vi "Pressure Temperature Monitor v3.vi"() -> ()   [LabVIEW 2016]
panel:
  in  "Gain":dbl=-10.0 format="%#_13g"
  in  "?":i32(ring)=2 items=["MKS 943 Cold Cathode"=1, "Thyracont All Range"=2]
  out "Pressure CH3":dbl=0.0007462942310144351 format="%#.2e"
  out "PRE Pressure 2":dbl(graph)=0.0007462942310144351
  in  "Gain":dbl=-10.0 format="%#_13g"
  in  "?":i32(ring)=1 items=["MKS 943 Cold Cathode"=1, "Thyracont All Range"=2]
  in  "?":i32(ring)=1 items=["MKS 943 Cold Cathode"=1, "Thyracont All Range"=2]
  in  "?":bool
  out "Pressure CH2":dbl=1.0051507111908389e-10 format="%#.2e"
  out "LL Pressure":dbl(graph)=1.0051507111908389e-10
  out "Tempreture CH2":dbl=3407.210278151436 format="%.1f"
  out "T2 Tempreture":dbl(graph)=3407.210278151436
  in  "Gain":dbl=-10.0 format="%#_13g"
  out "Tempreture CH1":dbl=21.38127177176258 format="%.1f"
  out "Pressure CH1":dbl=1.7008193334756893e-10 format="%#.2e"
  out "Heater Tempreture":dbl(graph)=21.38127177176258
  in  "?":bool
  out "Overdosing":bool
  in  "Dosing Limit":dbl=20.0 format="%#.2f"
  in  "Base Pressure":dbl=1e-10 format="%#.2e"
  out "PRE Pressure":dbl(graph)=1.7008193334756893e-10
  out "L":dbl=0.0047677960618811325 format="%.1e"
  in  "Pressure Limit":dbl=10.0 format="%#.2e"
  in  "?":bool
  # "Prep Pressure (Torr)"
  # "STM Pressure"
  # "LL Pressure"
  # "(Torr)"
  # "(Torr)"
  # "(Torr)"
  # "CH1 Temperature"
  # "CH2 Temperature"
  # "Langmuir"
  # "(°C )"
  # "(°C )"
  # "STM"
  # "PRE"
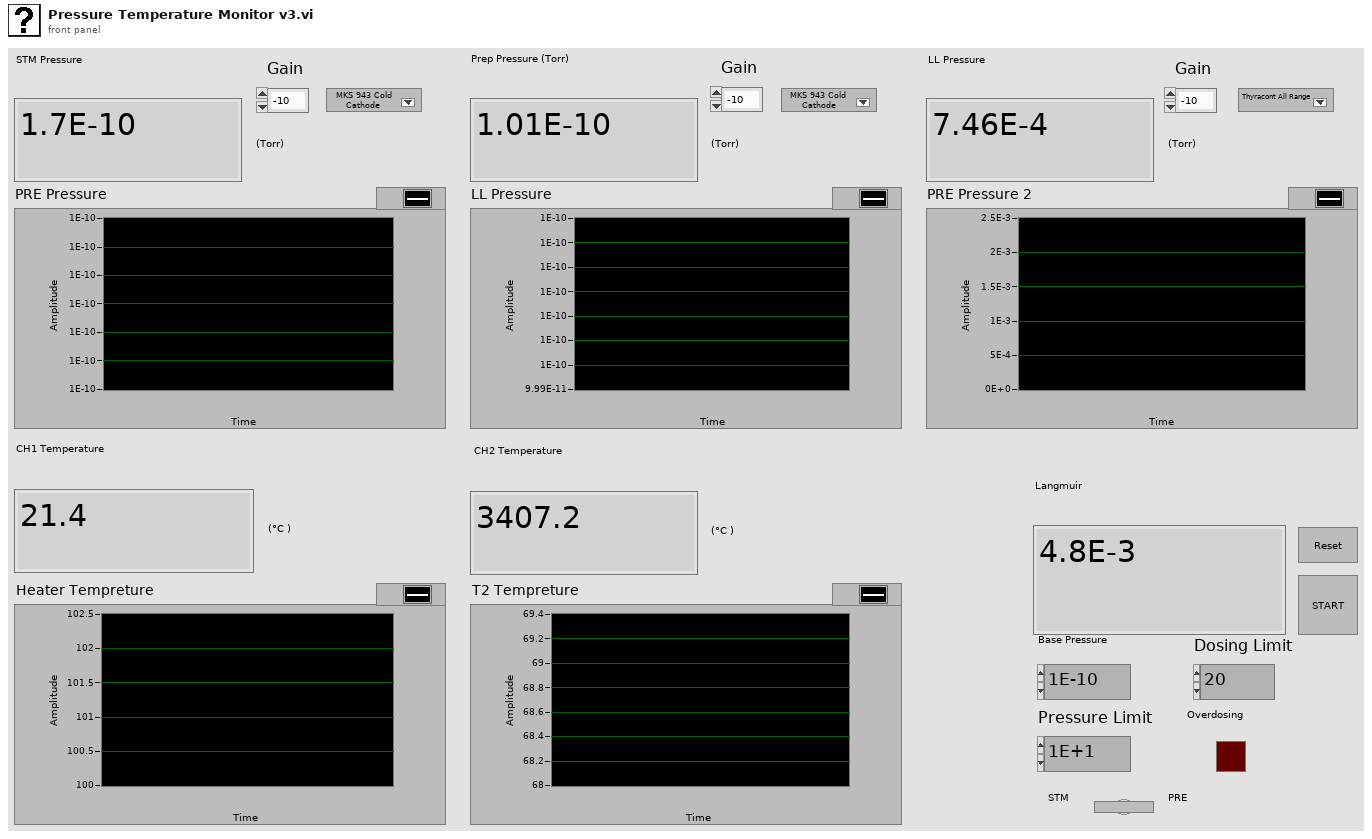
[diagram p1: front panel]
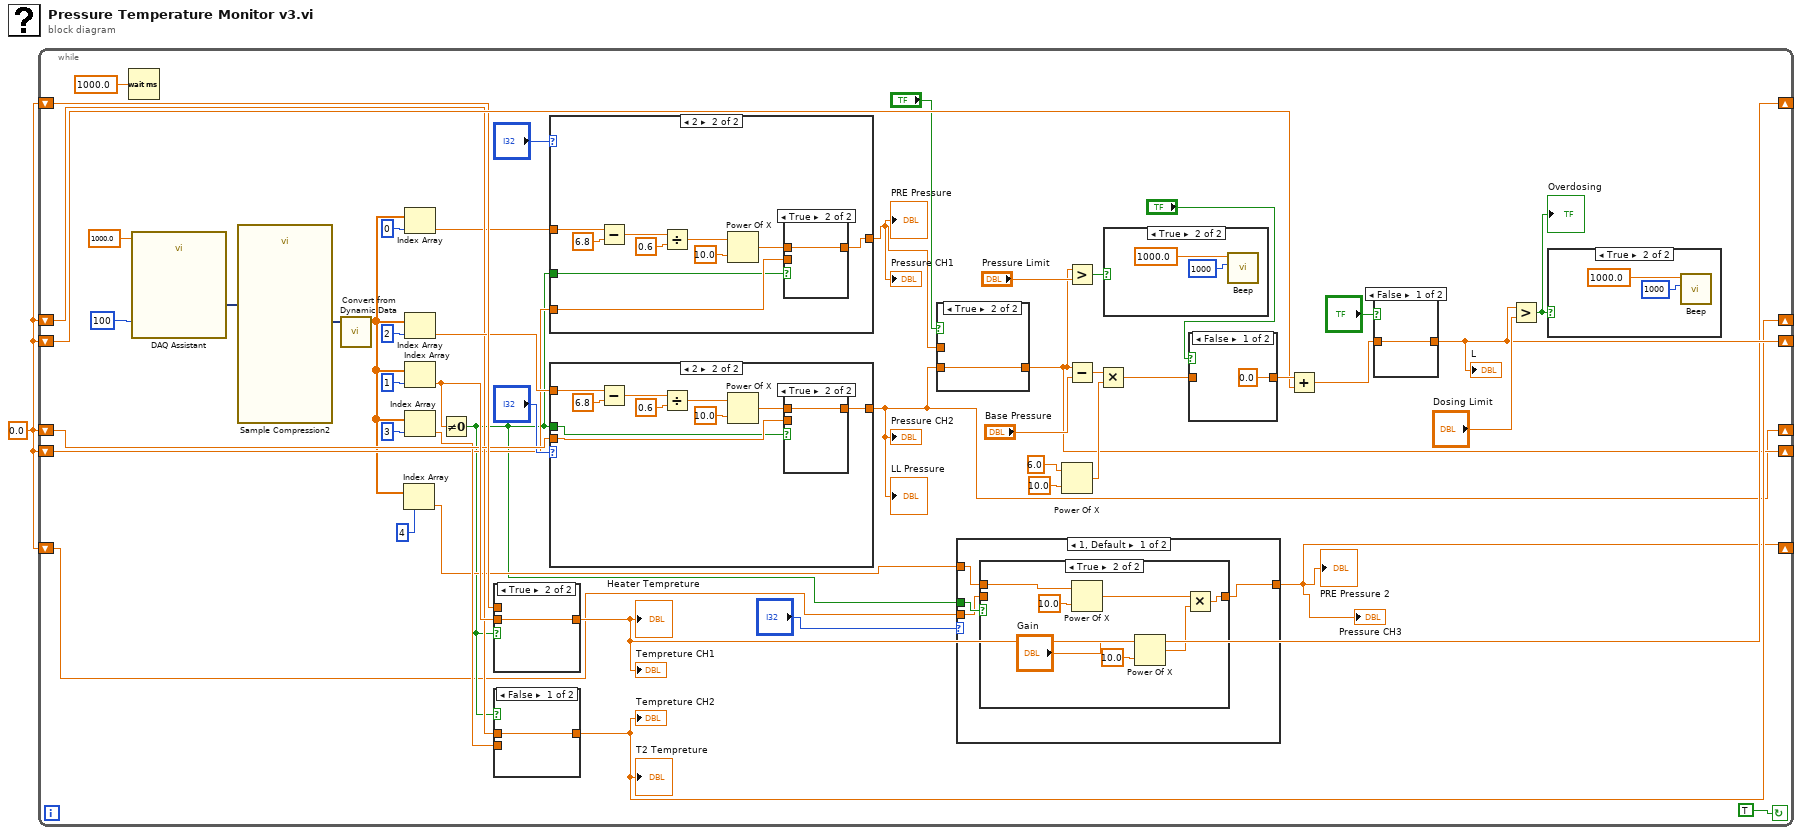
[diagram p0: block diagram]
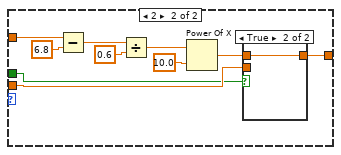
[diagram p3: hidden frame]
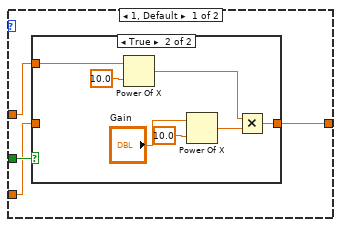
[diagram p5: hidden frame]
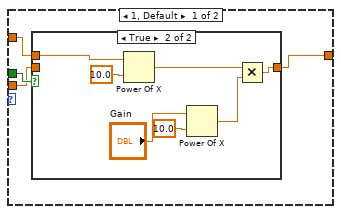
[diagram p8: hidden frame]
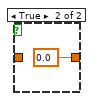
[diagram p14: hidden frame]
diagram:
  w1 = 0.0
  n1 = while {
    shift-left: w1 -> [w41]
    shift-right: [w39] -> _
    shift-right: [w15] -> _
    shift-left: w1 -> [w10]
    shift-right: [w33] -> _
    shift-left: w1 -> [w35]
    shift-right: [w13] -> _
    shift-left: w1 -> [w20]
    shift-right: [w17] -> _
    shift-left: w1 -> [w18]
    shift-right: [w2] -> _
    shift-left: w1 -> [w3]
    stop <- TRUE continue-if-true
    n2 = Wait (ms)(milliseconds to wait=1000.0 ("y")) -> ()  [unwired: 1 out]
    n3 = call "DAQ Assistant"("rate"=1000.0, "number of samples"=100) -> ("data"=w25:dynamicdata)  [unwired: 15 in, 2 out]
    n4 = call "Sample Compression2"("Signals"=w25) -> ("Mean"=w22:dynamicdata)  [unwired: 8 in, 2 out]
    n5 = call "Convert from Dynamic Data"("Dynamic Data Type"=w22) -> ("Array"=w7:dbl[])  [unwired: 3 in]
    n6 = Index Array(array=w7, index=4) -> (element=w6:dbl)
    n7 = Index Array(array=w7, index=0) -> (element=w12:dbl)
    n8 = Index Array(array=w7, index=2) -> (element=w21:dbl)
    n9 = Index Array(array=w7, index=1) -> (element=w34:dbl)
    n10 = Index Array(array=w7, index=3) -> (element=w19:dbl)
    n11 = Not Equal To 0?(x=w34) -> (x != 0?=w5:bool)
    n12 = case shown="True" w5 {
      tunnel: w34 -> [_ w128]
      tunnel: [w127 w128] -> w33
      tunnel: w35 -> [w127 _]
      frame False {
      }
      frame True {
      }
    }
    "Heater Tempreture" <- w33
    "Tempreture CH1" <- w33
    n13 = case shown="False" w5 {
      tunnel: w18 -> [w125 _]
      tunnel: [w125 w126] -> w17
      tunnel: w19 -> [_ w126]
      frame False {
      }
      frame True {
      }
    }
    "T2 Tempreture" <- w17
    "Tempreture CH2" <- w17
    n14 = case shown="2" "?" {
      tunnel: w5 -> [w78 w89]
      tunnel: w12 -> [w77 w88]
      tunnel: w10 -> [w76 w92]
      tunnel: [w75 w87] -> w9
      frame 1, Default {
        n15 = case shown="True" w78 {
          tunnel: w77 -> [_ w85]
          tunnel: [w79 w86] -> w75
          tunnel: w76 -> [w79 _]
          frame False {
          }
          frame True {
            n16 = Power Of X(1:10.0 ("x"), 2:w85) -> (0:w84:dbl)
            n17 = Power Of X(1:10.0 ("x"), 2:"Gain") -> (0:w82:dbl)
            n18 = Multiply(x=w84, y=w82) -> (x*y=w86:dbl)
          }
        }
      }
      frame 2 {
        n19 = Subtract(x=w88, y=6.8) -> (x-y=w94:dbl)
        n20 = Divide(x=w94, y=0.6) -> (x/y=w91:dbl)
        n21 = Power Of X(1:10.0 ("x"), 2:w91) -> (0:w90:dbl)
        n22 = case shown="True" w89 {
          tunnel: w90 -> [_ w98]
          tunnel: [w97 w98] -> w87
          tunnel: w92 -> [w97 _]
          frame False {
          }
          frame True {
          }
        }
      }
    }
    "PRE Pressure" <- w9
    "Pressure CH1" <- w9
    n23 = case shown="2" "?" {
      tunnel: w5 -> [w102 w112]
      tunnel: w21 -> [w101 w111]
      tunnel: w20 -> [w100 w115]
      tunnel: [w99 w116] -> w13
      frame 1, Default {
        n24 = case shown="True" w102 {
          tunnel: w101 -> [_ w109]
          tunnel: [w103 w110] -> w99
          tunnel: w100 -> [w103 _]
          frame False {
          }
          frame True {
            n25 = Power Of X(1:10.0 ("x"), 2:w109) -> (0:w108:dbl)
            n26 = Power Of X(1:10.0 ("x"), 2:"Gain") -> (0:w106:dbl)
            n27 = Multiply(x=w108, y=w106) -> (x*y=w110:dbl)
          }
        }
      }
      frame 2 {
        n28 = Subtract(x=w111, y=6.8) -> (x-y=w118:dbl)
        n29 = Divide(x=w118, y=0.6) -> (x/y=w114:dbl)
        n30 = Power Of X(1:10.0 ("x"), 2:w114) -> (0:w113:dbl)
        n31 = case shown="True" w112 {
          tunnel: w113 -> [_ w122]
          tunnel: [w121 w122] -> w116
          tunnel: w115 -> [w121 _]
          frame False {
          }
          frame True {
          }
        }
      }
    }
    "LL Pressure" <- w13
    "Pressure CH2" <- w13
    n32 = case shown="True" "?" {
      tunnel: w9 -> [w123 _]
      tunnel: [w123 w124] -> w15
      tunnel: w13 -> [_ w124]
      frame False {
      }
      frame True {
      }
    }
    n33 = case shown="1, Default" "?" {
      tunnel: w5 -> [w54 w64]
      tunnel: w6 -> [w53 w63]
      tunnel: w3 -> [w52 w67]
      tunnel: [w51 w68] -> w2
      frame 1, Default {
        n34 = case shown="True" w54 {
          tunnel: w53 -> [_ w61]
          tunnel: [w55 w62] -> w51
          tunnel: w52 -> [w55 _]
          frame False {
          }
          frame True {
            n35 = Power Of X(1:10.0 ("x"), 2:w61) -> (0:w60:dbl)
            n36 = Power Of X(1:10.0 ("x"), 2:"Gain") -> (0:w58:dbl)
            n37 = Multiply(x=w60, y=w58) -> (x*y=w62:dbl)
          }
        }
      }
      frame 2 {
        n38 = Subtract(x=w63, y=6.8) -> (x-y=w70:dbl)
        n39 = Divide(x=w70, y=0.6) -> (x/y=w66:dbl)
        n40 = Power Of X(1:10.0 ("x"), 2:w66) -> (0:w65:dbl)
        n41 = case shown="True" w64 {
          tunnel: w65 -> [_ w74]
          tunnel: [w73 w74] -> w68
          tunnel: w67 -> [w73 _]
          frame False {
          }
          frame True {
          }
        }
      }
    }
    "PRE Pressure 2" <- w2
    "Pressure CH3" <- w2
    n42 = Power Of X(1:10.0 ("x"), 2:6.0 ("y")) -> (0:w29:dbl)
    n43 = Greater?(x=w15, y="Pressure Limit") -> (0:w49:bool)
    n44 = Subtract(x=w15, y="Base Pressure") -> (x-y=w32:dbl)
    n45 = Multiply(x=w32, y=w29) -> (x*y=w28:dbl)
    n46 = case shown="True" w49 {
      frame False {
      }
      frame True {
        n47 = call <vilib>:"Beep.vi"("duration (msec)"=i16 1000 ("duration (msec) - ignored"), "frequency (Hz)"=1000.0 ("frequency (Hz) - ignored")) -> ()  [unwired: 10 in]
      }
    }
    n48 = case shown="False" "?" {
      tunnel: [0.0 w134] -> w42
      tunnel: w28 -> [_ w134]
      frame False {
      }
      frame True {
      }
    }
    n49 = Add(x=w42, y=w41) -> (x+y=w40:dbl)
    n50 = case shown="False" "?" {
      tunnel: w40 -> [w129 _]
      tunnel: [w129 0.0 ("y")] -> w39
      frame False {
      }
      frame True {
      }
    }
    "L" <- w39
    n51 = Greater?(x=w39, y="Dosing Limit") -> (0:w43:bool)
    "Overdosing" <- w43
    n52 = case shown="True" w43 {
      frame False {
      }
      frame True {
        n53 = call <vilib>:"Beep.vi"("duration (msec)"=i16 1000 ("duration (msec) - ignored"), "frequency (Hz)"=1000.0 ("frequency (Hz) - ignored")) -> ()  [unwired: 10 in]
      }
    }
  }
